vi "pumpSwitch.vi"(8 "error in (no error)":errorcluster, 10 "Sensors":refnum<class "Sensor.lvclass">[](array[class]), 11 "Pump in":refnum<class "Pump.lvclass">) -> (0 "error out":errorcluster, 3 "Pump out":refnum<class "Pump.lvclass">)   [LabVIEW 2018, in "Pump.lvclass"]
uses:
  Pump.lvclass
  Sensor Class/Sensor.lvclass
  Pump.lvclass/Pump.ctl
  Sensor Class/Sensor.lvclass/Sensor.ctl
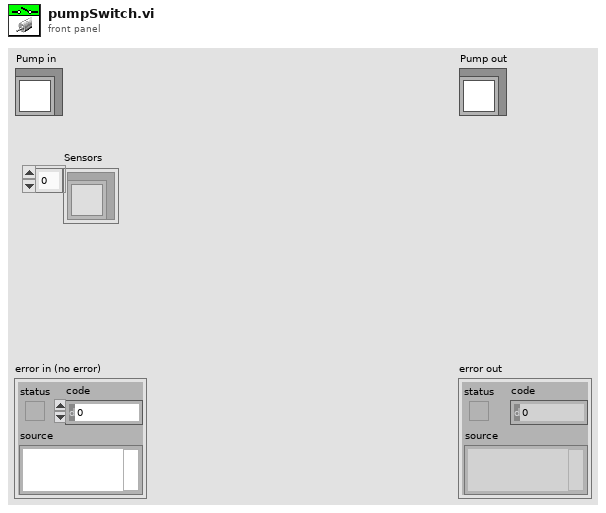
[diagram p1: front panel]
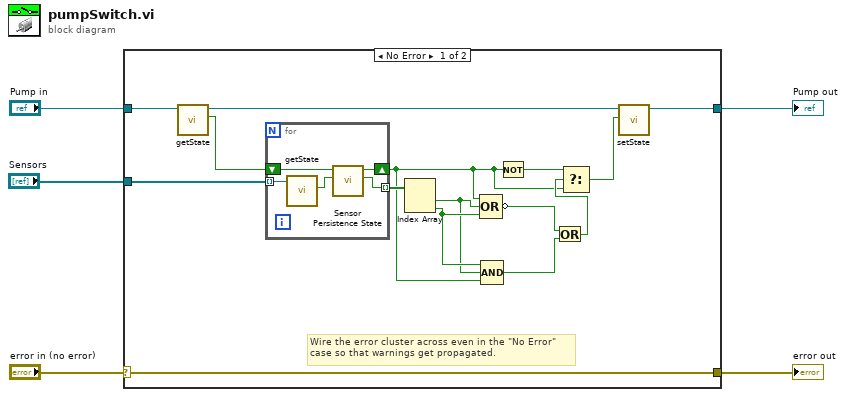
[diagram p0: block diagram]
diagram:
  n1 = case shown="No Error" "error in (no error)" {
    selector: "error in (no error)" -> [w20 w27]
    tunnel: [w20 w27] -> w4
    tunnel: [w16 w26] -> w2
    tunnel: "Pump in" -> [w18 w26]
    tunnel: "Sensors" -> [w19 _]
    frame No Error {
      # "Wire the error cluster across even in the \"No Error\"\ncase so that warnings get propagated."
      n2 = call "getState.vi"("Pump in"=w18) -> ("state"=w15:bool, "Pump out"=w17:refnum<class "Pump.lvclass">)  [unwired: 8 in, 1 out]
      n3 = for {
        tunnel: w19 -> [w25] mode=indexing
        tunnel: [w23] -> w14 mode=indexing
        shift-right: [w21] -> w6
        shift-left: w15 -> [w22]
        n4 = call "getState.vi"("Sensor in"=w25) -> ("State"=w24:bool)  [unwired: 8 in, 2 out]
        n5 = call "Sensor Persistence State.vi"("Sensor"=w24, "Pump State in"=w22) -> ("Persistent State"=w23:bool, "Pump State out"=w21:bool)  [unwired: 8 in]
      }
      n6 = Index Array(array=w14) -> (element #1=w8:bool, element #2=w9:bool)  [unwired: 2 in]
      n7 = Compound Arithmetic op=OR(w6, w8, w9) -> (invert w11:bool)
      n8 = Compound Arithmetic op=AND(w9, w8, w6) -> (w10:bool)
      n9 = Not(x=w6) -> (.not. x?=w13:bool)
      n10 = Or(x=w11, y=w10) -> (x .or. y?=w7:bool)
      n11 = Select(t=w13, s=w7, f=w6) -> (s? t:f=w12:bool)
      n12 = call "setState.vi"("state"=w12, "Pump in"=w17) -> ("Pump out"=w16:refnum<class "Pump.lvclass">)  [unwired: 8 in, 1 out]
    }
    frame Error {
    }
  }
  "error out" <- w4
  "Pump out" <- w2
